vi "Ethernet Find Message Names&Max Index.vi"(8 "error in":errorcluster, 11 "Frame Info":T1[](array[typedef])) -> (0 "error out":errorcluster, 2 "Dynamic column":i32[][](array[numeric]), 3 "Dynamic Message":string[](array[string]))   [LabVIEW 2024]
doc: "All Rights Reserved © 2017 SyncSols"
uses:
  Controls/Ethernet Frame Info Cluster.ctl
  Controls/Ethernet Message Info Cluster.ctl
  Controls/Ethernet Dynamic Data Cluster.ctl
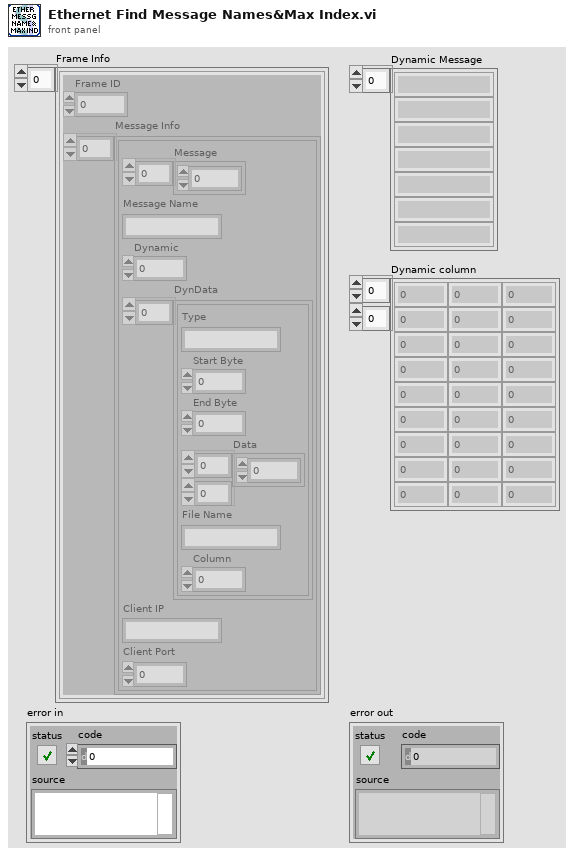
[diagram p1: front panel]
types:
  T1 = typedef "Ethernet Frame Info Cluster.ctl" = cluster{"Frame ID":u16, "Message Info":T2[]}
  T2 = typedef "Ethernet Message Info Cluster.ctl" = cluster{"Message":u8[], "Message Name":string, "Dynamic":u8, "DynData":T3[], "Client IP":string, "Client Port":u16}
  T3 = typedef "Ethernet Dynamic Data Cluster.ctl" = cluster{"Type":string, "Start Byte":u8, "End Byte":u8, "Data":u32[][], "File Name":string, "Column":i32}
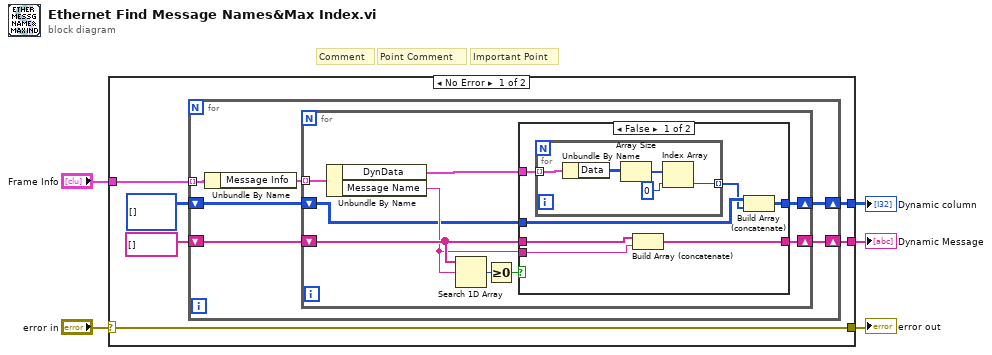
[diagram p0: block diagram]
diagram:
  # "Important Point"
  # "Point Comment"
  # "Comment"
  n1 = case shown="No Error" "error in" {
    selector: "error in" -> [w11 w41]
    tunnel: [w11 w41] -> w3
    tunnel: "Frame Info" -> [w10 _]
    tunnel: [w7 _] -> w2
    tunnel: [w6 _] -> w1
    frame No Error {
      n2 = for {
        tunnel: w10 -> [w17] mode=indexing
        shift-right: [w13] -> w6
        shift-left: i32[][] [] -> [w14]
        shift-right: [w15] -> w7
        shift-left: string[] [] -> [w12]
        n3 = Unbundle By Name(w17) -> ("Message Info"=w16:T2[])
        n4 = for {
          tunnel: w16 -> [w26] mode=indexing
          shift-right: [w25] -> w15
          shift-left: w12 -> [w24]
          shift-right: [w19] -> w13
          shift-left: w14 -> [w18]
          n5 = Unbundle By Name(w26) -> ("DynData"=w20:T3[], "Message Name"=w21:string)
          n6 = Search 1D Array(1D array=w24, element=w21) -> (index of element=w23:i32)  [unwired: 1 in]
          n7 = Greater Or Equal To 0?(x=w23) -> (x >= 0?=w22:bool)
          n8 = case shown="False" w22 {
            tunnel: w21 -> [w33 _]
            tunnel: [w32 w40] -> w25
            tunnel: w24 -> [w31 w40]
            tunnel: w20 -> [w30 _]
            tunnel: [w29 w39] -> w19
            tunnel: w18 -> [w28 w39]
            frame False {
              n9 = for {
                tunnel: w30 -> [w38] mode=indexing
                tunnel: [w35] -> w27 mode=indexing
                n10 = Unbundle By Name(w38) -> ("Data"=w37:u32[][])
                n11 = Array Size(array=w37) -> (size(s)=w36:i32[])
                n12 = Index Array(array=w36, index=0) -> (element=w35:i32)
              }
              n13 = Build Array (concatenate)(w31, w33) -> (w32:string[])
              n14 = Build Array (concatenate)(w28, w27) -> (w29:i32[][])
            }
            frame True {
            }
          }
        }
      }
    }
    frame Error {
    }
  }
  "error out" <- w3
  "Dynamic Message" <- w2
  "Dynamic column" <- w1
